vi "Control_Panel_Begin.vi"   [LabVIEW 2019]
uses:
  Control_Panel_Cluster.ctl
  Control_Panel_States.ctl
  Control_Panel_Globals.vi
types:
  T1 = typedef "Control_Panel_Cluster.ctl" = cluster{"Control_State":T2, "Start_Movement":bool, "Abort":bool, "Rotation_Control?":bool, "Positional_Control? ":bool, "Throttle":dbl, "Extend?":bool}
  T2 = typedef "Control_Panel_States.ctl" = enum16{"No-Op", "Rotational_Control", "Positional_Control", "Manual_Control"}
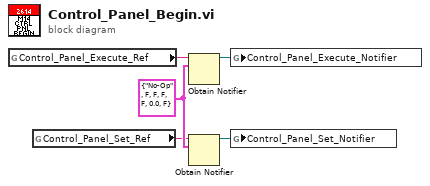
[diagram p0: block diagram]
diagram:
  w4 = T1 {"Control_State"=enum."No-Op", "Start_Movement"=FALSE, "Abort"=FALSE, "Rotation_Control?"=FALSE, "Positional_Control? "=FALSE, "Throttle"=0.0, "Extend?"=FALSE} ("Control_Panel_Cluster")
  n1 = global read "Control_Panel_Globals.vi" "Control_Panel_Execute_Ref"() -> (w5:string)
  n2 = global read "Control_Panel_Globals.vi" "Control_Panel_Set_Ref"() -> (w3:string)
  n3 = Obtain Notifier(name (unnamed)=w5, notification data type=w4) -> (notifier out=w2:refnum<notifier>)  [unwired: 2 in, 2 out]
  n4 = Obtain Notifier(name (unnamed)=w3, notification data type=w4) -> (notifier out=w1:refnum<notifier>)  [unwired: 2 in, 2 out]
  n5 = global write "Control_Panel_Globals.vi" "Control_Panel_Execute_Notifier"(w2) -> ()
  n6 = global write "Control_Panel_Globals.vi" "Control_Panel_Set_Notifier"(w1) -> ()
